vi "read hi scores.vi"(8 "Error In":errorcluster, 11 "file path (dialog if empty)":path) -> (0 "Error Out":errorcluster, 2 "Lowest Score":i64, 3 "Score Array Out":T1[](array[typedef]))   [LabVIEW 2017]
uses:
  controls/scores.ctl
  <vilib>/Utility/file.llb/Read From Spreadsheet File (I64).vi
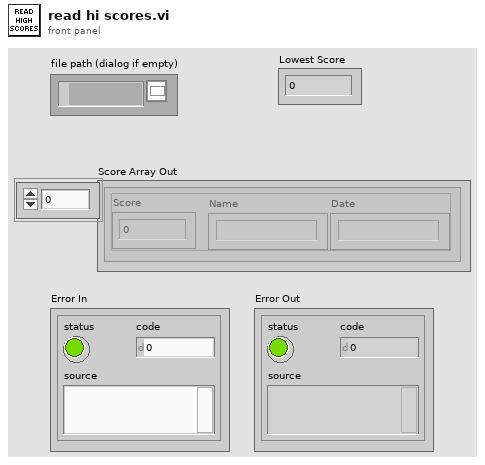
[diagram p1: front panel]
types:
  T1 = typedef "scores.ctl" = cluster{"Score":dbl, "Name":string, "Date":string}
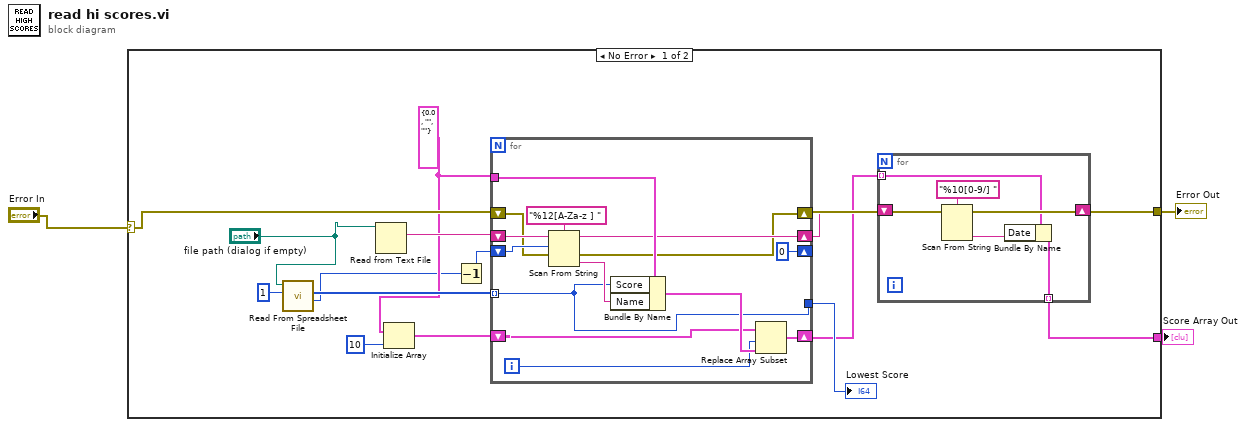
[diagram p0: block diagram]
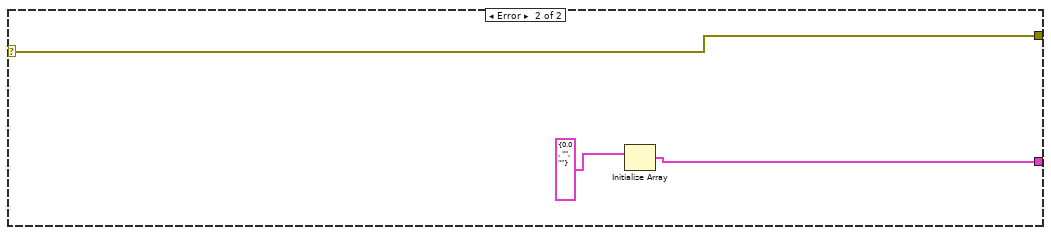
[diagram p2: hidden frame]
diagram:
  n1 = case shown="No Error" "Error In" {
    selector: "Error In" -> [w12 w41]
    tunnel: [w6 w39] -> w3
    tunnel: [w11 w41] -> w1
    frame No Error {
      w8 = T1 {"Score"=0.0, "Name"="", "Date"=""} ("Scores")
      n2 = call-poly <vilib>:"Read From Spreadsheet File.vi"("number of rows (all:-1)"=1, "file path (dialog if empty)"="file path (dialog if empty)") -> ("mark after read (chars.)"=w4:i32, "first row"=w16:i64[])  [unwired: 5 in, 3 out]
      n3 = Read from Text File(file (use dialog)="file path (dialog if empty)") -> (text=w17:string)  [unwired: 3 in, 3 out]
      n4 = Initialize Array(w8, 10 ("dimension size")) -> (w14:T1[])
      n5 = Decrement(x=w4) -> (x-1=w13:i32)
      n6 = for {
        tunnel: w8 -> [w37]
        tunnel: w16 -> [w25] mode=indexing
        shift-right: [0 ("mark after read (chars.)")] -> _
        shift-left: w13 -> [w29]
        shift-right: [w31] -> w5
        shift-left: w17 -> [w38]
        shift-right: [w26] -> w7
        shift-left: w14 -> [w34]
        tunnel: [w25] -> w9
        shift-right: [w27] -> w11
        shift-left: w12 -> [w28]
        i -> [w33]
        n7 = Scan From String(format string="%12[A-Za-z ] ", input string=w38, initial scan location=w29, error in=w28) -> (remaining string=w31:string, error out=w27:errorcluster, output 1=w32:string)  [unwired: 1 in, 1 out]
        n8 = Bundle By Name(cluster=w37, "Score"=w25, "Name"=w32) -> (w35:T1)
        n9 = Replace Array Subset(array=w34, new element=w35, index=w33) -> (w26:T1[])
      }
      "Lowest Score" <- w9
      n10 = for {
        tunnel: w7 -> [w24] mode=indexing
        tunnel: [w23] -> w6 mode=indexing
        shift-right: [w20] -> _
        shift-left: w5 -> [w21]
        n11 = Scan From String(format string="%10[0-9/] ", input string=w21) -> (remaining string=w20:string, output 1=w19:string)  [unwired: 3 in, 2 out]
        n12 = Bundle By Name(cluster=w24, "Date"=w19) -> (w23:T1)
      }
    }
    frame Error {
      n13 = Initialize Array(T1 {"Score"=0.0, "Name"="", "Date"=""} ("Scores")) -> (w39:T1[])  [unwired: 1 in]
    }
  }
  "Score Array Out" <- w3
  "Error Out" <- w1
